vi "FTW-Publisher-Listener-Start.vi"(0 "FTW Publisher in":refnum<class "FTW-Publisher.lvclass">, 5 "Send Timeout":i32, 7 "Send Buffer Depth":i32, 11 "error in (no error)":errorcluster) -> (4 "FTW Publisher out":refnum<class "FTW-Publisher.lvclass">, 15 "error out":errorcluster)   [LabVIEW 2013, in "FTW-Publisher.lvclass"]
uses:
  FTW-Publisher.lvclass
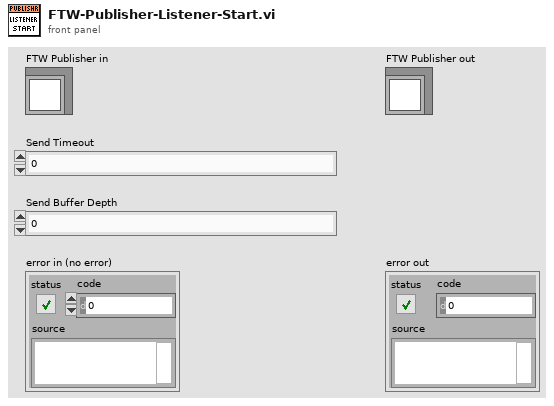
[diagram p1: front panel]
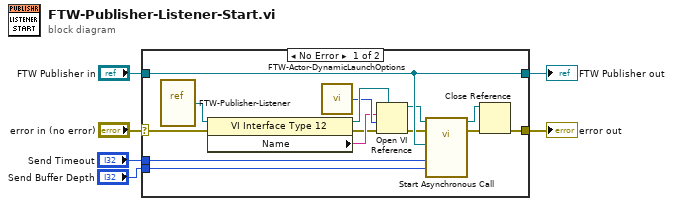
[diagram p0: block diagram]
diagram:
  n1 = case shown="No Error" "error in (no error)" {
    selector: "error in (no error)" -> [w19 w21]
    tunnel: [w20 w22] -> w6
    tunnel: "FTW Publisher in" -> [w20 w22]
    tunnel: "Send Buffer Depth" -> [w18 _]
    tunnel: "Send Timeout" -> [w17 _]
    tunnel: [w15 w21] -> w1
    frame No Error {
      n2 = vi-ref "FTW-Publisher-Listener.vi"() -> (w7:refnum<vi>)
      n3 = property class="VI Interface Type 12"(reference=w7, error in=w19) -> (reference out=w11:refnum<vi>, error out=w8:errorcluster, "Name"=w9:string)
      n4 = call "FTW-Actor-DynamicLaunchOptions.vi"() -> ("Open VI Ref Options"=w10:i32)
      n5 = Open VI Reference(type specifier VI Refnum (for type only)=w11, vi path=w9, options=w10, error in (no error)=w8) -> (vi reference=w13:refnum<vi>, error out=w16:errorcluster)  [unwired: 2 in]
      n6 = call-by-ref "Start Asynchronous Call"(reference=w13, error in=w16, "keep most recent"=w18, "Timeout"=w17, "FTW Publisher"=w20) -> (reference out=w14:refnum<vi>, error out=w12:errorcluster)  [unwired: 2 in]
      n7 = Close Reference(reference=w14, error in (no error)=w12) -> (error out=w15:errorcluster)
    }
    frame Error {
    }
  }
  "FTW Publisher out" <- w6
  "error out" <- w1
